vi "Read content-encoding.vi"(8 "error in (no error)":errorcluster, 11 "TCPPacket in":refnum<class "TCPPacket.lvclass">) -> (0 "error out":errorcluster, 2 "content-encoding":string, 3 "TCPPacket out":refnum<class "TCPPacket.lvclass">)   [LabVIEW 2019, in "TCPPacket.lvclass"]
uses:
  TCPPacket.lvclass
  TCPPacket.lvclass/TCPPacket.ctl
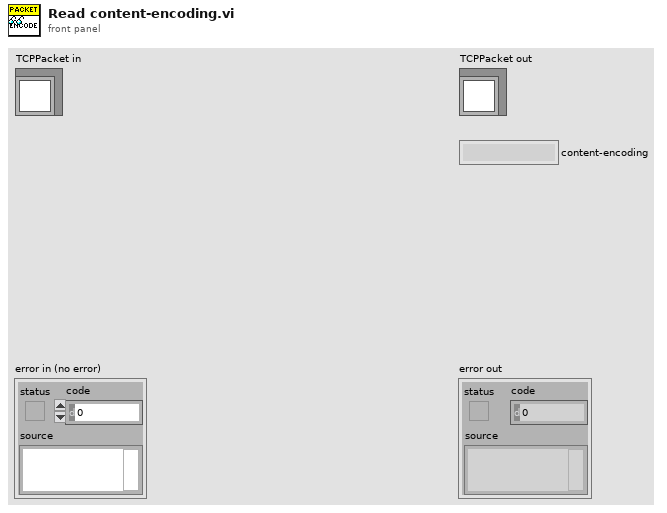
[diagram p1: front panel]
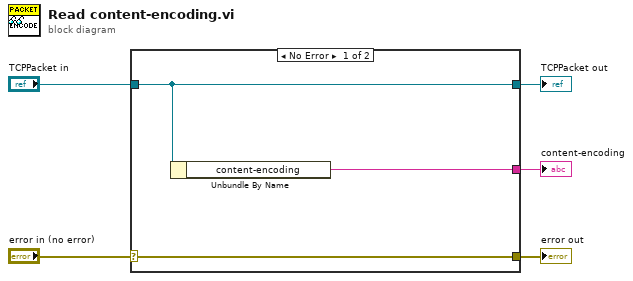
[diagram p0: block diagram]
diagram:
  n1 = case shown="No Error" "error in (no error)" {
    selector: "error in (no error)" -> [w8 w9]
    tunnel: [w8 w9] -> w4
    tunnel: [w7 w10] -> w2
    tunnel: "TCPPacket in" -> [w7 w10]
    tunnel: [w6 _] -> w1
    frame No Error {
      n2 = Unbundle By Name(w7) -> ("content-encoding"=w6:string)
    }
    frame Error {
    }
  }
  "error out" <- w4
  "TCPPacket out" <- w2
  "content-encoding" <- w1
